vi "Text_File.vi"   [LabVIEW 2024, in "Launcher_DTU.lvlib"]
uses:
  Launcher_DTU.lvlib
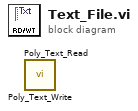
[diagram p0: block diagram]
diagram:
  n1 = call "Poly_Text_Write.vi"() -> ()  [unwired: 11 in, 1 out]
  n2 = call "Poly_Text_Read.vi"() -> ()  [unwired: 10 in, 2 out]
